vi "Read Digital.vi"(8 "error in (no error)":errorcluster, 10 "Params":variant, 11 "NI Digital Input in":refnum<class "NI Digital Input.lvclass">) -> (0 "error out":errorcluster, 2 "Data":variant, 3 "NI Digital Input out":refnum<class "NI Digital Input.lvclass">)   [LabVIEW 2020, in "NI DAQmx.lvlib" / "NI Digital Input.lvclass"]
uses:
  NI Digital Input.lvclass
  D:/WSGitHub/RTFWK/Realization/NI DAQmx Base/NI DAQmx Base.lvclass
  <vilib>/DAQmx/read.llb/DAQmx Read (Digital 1D U32 1Chan NSamp).vi
  <vilib>/DAQmx/read.llb/DAQmx Read (Digital U32 1Chan 1Samp).vi
  <vilib>/DAQmx/read.llb/DAQmx Read (Digital 2D U32 NChan NSamp).vi
  <vilib>/DAQmx/read.llb/DAQmx Read (Digital 1D U32 NChan 1Samp).vi
  <vilib>/DAQmx/miscellaneous.llb/DAQmx Fill In Error Info.vi
  <resource>/objmgr/daqmx.rc
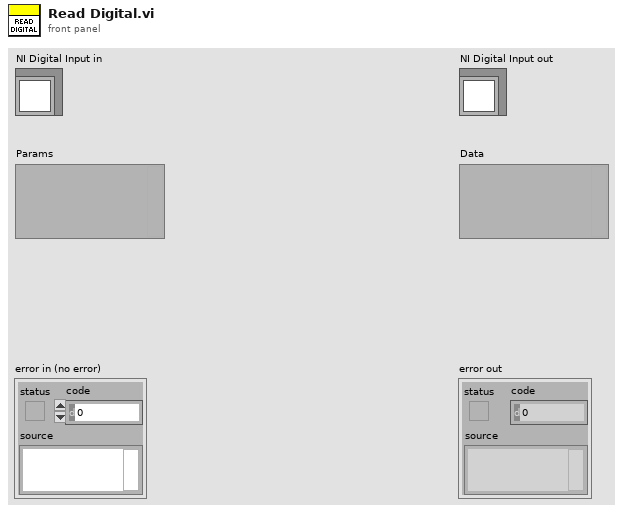
[diagram p1: front panel]
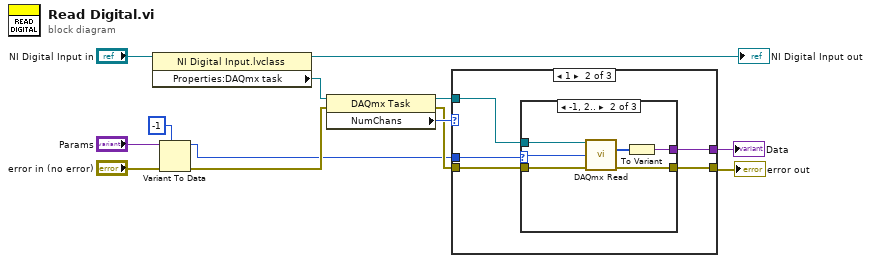
[diagram p0: block diagram]
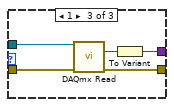
[diagram p4: hidden frame]
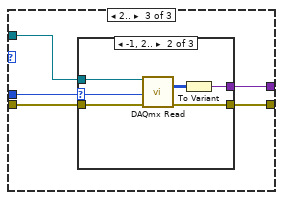
[diagram p5: hidden frame]
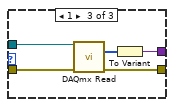
[diagram p7: hidden frame]
diagram:
  n1 = property class="NI Digital Input.lvclass"(reference="NI Digital Input in") -> (reference out=→"NI Digital Input out":refnum<class "NI Digital Input.lvclass">, "Properties:DAQmx task"=w6:refnum<k21>)  [unwired: 1 in, 1 out]
  n2 = Variant To Data(error in="error in (no error)", type=-1 ("number of samples per channel"), Variant="Params") -> (data=w3:i32, error out=w8:errorcluster)
  n3 = property class="DAQmx Task"(reference=w6, error in=w8) -> (reference out=w4:refnum<k21>, error out=w5:errorcluster, "NumChans"=w7:u32)
  n4 = case shown="1" w7 {
    tunnel: [w14 w18 w35] -> w1
    tunnel: w5 -> [w14 w19 w36]
    tunnel: w4 -> [_ w17 w34]
    tunnel: [_ w16 w33] -> w2
    tunnel: w3 -> [_ w15 w32]
    frame 0, Default {
    }
    frame 1 {
      n5 = case shown="-1, 2.." w15 {
        selector: w15 -> [_ w21 _]
        tunnel: w19 -> [w20 w26 w31]
        tunnel: [w20 w25 w30] -> w18
        tunnel: w17 -> [_ w24 w29]
        tunnel: [_ w22 w27] -> w16
        frame 0, Default {
        }
        frame -1, 2.. {
          n6 = call-poly <vilib>:"DAQmx Read.vi"("task/channels in"=w24, "number of samples per channel"=w21, "error in"=w26) -> ("data"=w23:u32[], "error out"=w25:errorcluster)  [unwired: 10 in, 1 out]
          n7 = To Variant(anything=w23) -> (Variant=w22:variant)
        }
        frame 1 {
          n8 = call-poly <vilib>:"DAQmx Read.vi"("task/channels in"=w29, "error in"=w31) -> ("data"=w28:u32, "error out"=w30:errorcluster)  [unwired: 11 in, 1 out]
          n9 = To Variant(anything=w28) -> (Variant=w27:variant)
        }
      }
    }
    frame 2.. {
      n10 = case shown="-1, 2.." w32 {
        selector: w32 -> [_ w38 _]
        tunnel: w36 -> [w37 w43 w48]
        tunnel: [w37 w42 w47] -> w35
        tunnel: w34 -> [_ w41 w46]
        tunnel: [_ w39 w44] -> w33
        frame 0, Default {
        }
        frame -1, 2.. {
          n11 = call-poly <vilib>:"DAQmx Read.vi"("task/channels in"=w41, "number of samples per channel"=w38, "error in"=w43) -> ("data"=w40:u32[][], "error out"=w42:errorcluster)  [unwired: 10 in, 1 out]
          n12 = To Variant(anything=w40) -> (Variant=w39:variant)
        }
        frame 1 {
          n13 = call-poly <vilib>:"DAQmx Read.vi"("task/channels in"=w46, "error in"=w48) -> ("data"=w45:u32[], "error out"=w47:errorcluster)  [unwired: 11 in, 1 out]
          n14 = To Variant(anything=w45) -> (Variant=w44:variant)
        }
      }
    }
  }
  "error out" <- w1
  "Data" <- w2
